vi "Init.vi"(8 "error in (no error)":errorcluster, 10 "App":refnum<class "App.lvclass">) -> (0 "error out":errorcluster, 3 "VolatusCore out":refnum<class "VolatusCoreTask.lvclass">)   [LabVIEW 2020, in "Volatus.lvlib" / "VolatusCoreTask.lvclass"]
uses:
  VolatusCoreTask.lvclass
  App/App.lvclass
  VolatusCoreTask.lvclass/VolatusCoreTask.ctl
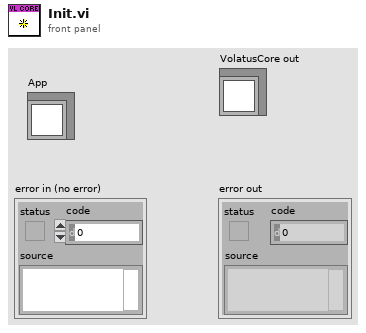
[diagram p1: front panel]
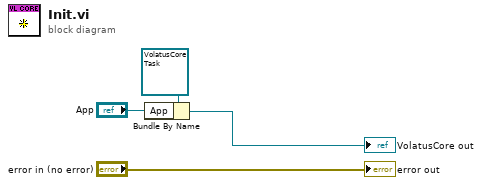
[diagram p0: block diagram]
diagram:
  n1 = Bundle By Name(cluster=refnum<class "VolatusCoreTask.lvclass"> refnum ("VolatusCore in"), "App"="App") -> (→"VolatusCore out":refnum<class "VolatusCoreTask.lvclass">)
  "error out" <- "error in (no error)"
